vi "temp Server.vi"() -> ()   [LabVIEW 2020]
panel:
  in  "Iteration Rate":u32=500
  out "Heater":bool
  in  "stop":bool
  out "Thermometer":dbl(slide) scale=0.0..100.0
  out "Waveform Chart":dynamicdata(graph)
  in  "Min Temp Limit":dbl(knob)=40.0 scale=40.0..60.0
  in  "Max Temp Limit":dbl(knob)=70.0 scale=60.0..80.0
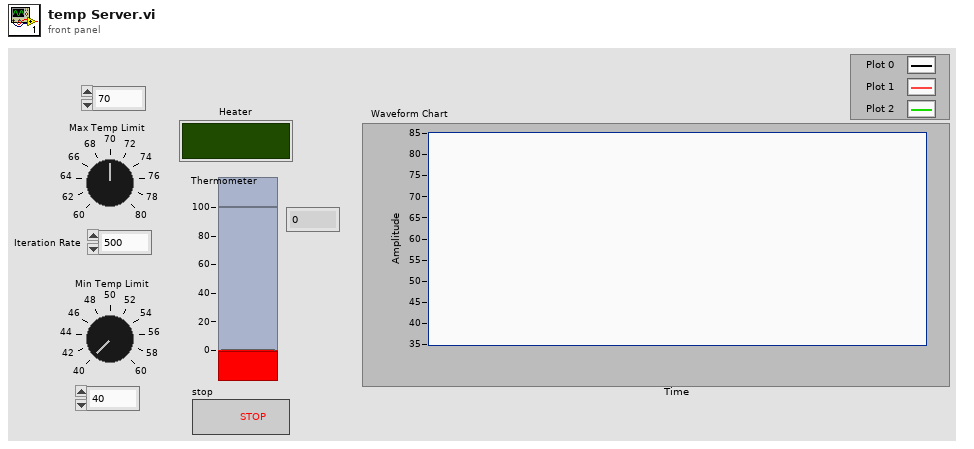
[diagram p1: front panel]
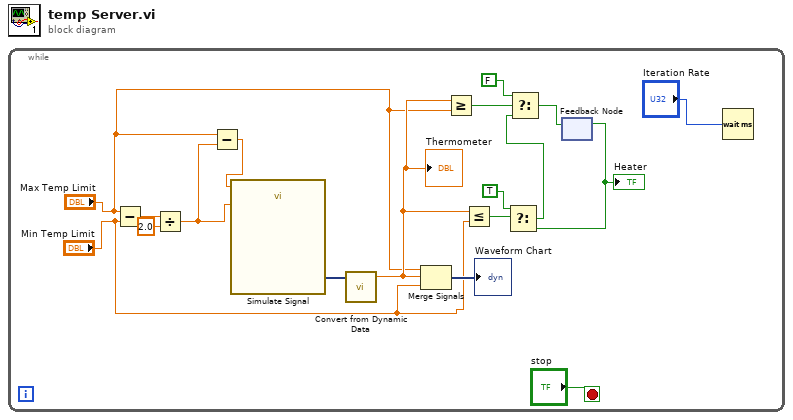
[diagram p0: block diagram]
diagram:
  n1 = while {
    stop <- "stop" stop-if-true
    n2 = Subtract(x="Max Temp Limit", y="Min Temp Limit") -> (x-y=w18:dbl)
    n3 = Divide(x=w18, y=2.0) -> (x/y=w16:dbl)
    n4 = Subtract(x="Max Temp Limit", y=w16) -> (x-y=w15:dbl)
    n5 = call "Simulate Signal"("Offset"=w15, "Amplitude"=w16) -> ("Sine with Uniform Noise"=w14:dynamicdata)  [unwired: 12 in, 1 out]
    n6 = call "Convert from Dynamic Data"("Dynamic Data Type"=w14) -> ("Scalar"=w4:dbl)  [unwired: 3 in]
    "Thermometer" <- w4
    n7 = Merge Signals("Max Temp Limit", w4, "Min Temp Limit") -> (→"Waveform Chart":dynamicdata)
    n8 = Greater Or Equal?(x=w4, y="Max Temp Limit") -> (x >= y?=w11:bool)
    n9 = Less Or Equal?(x=w4, y="Min Temp Limit") -> (x <= y?=w3:bool)
    n10 = feedback #1() -> (w6:bool)  [unwired: 1 in]
    "Heater" <- w6
    n11 = Select(t=TRUE, s=w3, f=w6) -> (s? t:f=w8:bool)
    n12 = Select(t=FALSE, s=w11, f=w8) -> (s? t:f=w7:bool)
    n13 = feedback-in #1(w7) -> ()
    n14 = Wait (ms)(milliseconds to wait="Iteration Rate") -> ()  [unwired: 1 out]
  }
